vi "FpgaSession_GET.vi"(8 "error in":errorcluster, 11 "lia rt in":refnum<class "Lock-In Amplifier Example RT.lvclass">) -> (0 "error out":errorcluster, 2 "fpga interface":refnum<class "LIA Host Interface FPGA.lvclass">, 3 "lia rt out":refnum<class "Lock-In Amplifier Example RT.lvclass">)   [LabVIEW 2017, in "Lock-In Amplifier Example RT.lvclass"]
uses:
  Lock-In Amplifier Example RT.lvclass
  interface/Interface FPGA/LIA Host Interface FPGA.lvclass
  Lock-In Amplifier Example RT.lvclass/Lock-In Amplifier Example RT.ctl
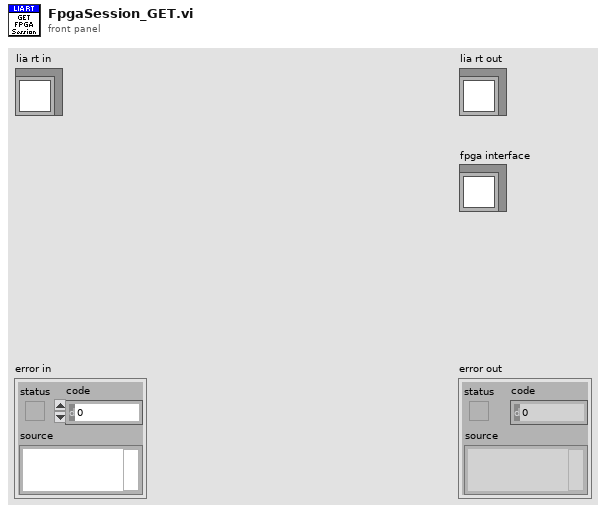
[diagram p1: front panel]
types:
  T1 = typedef "Lock-In Amplifier Example RT.lvclass/session data.ctl" = cluster{"server":refnum<class "RT FlexRIO Server TCP.lvclass">, "fpga interface":refnum<class "LIA Host Interface FPGA.lvclass">}
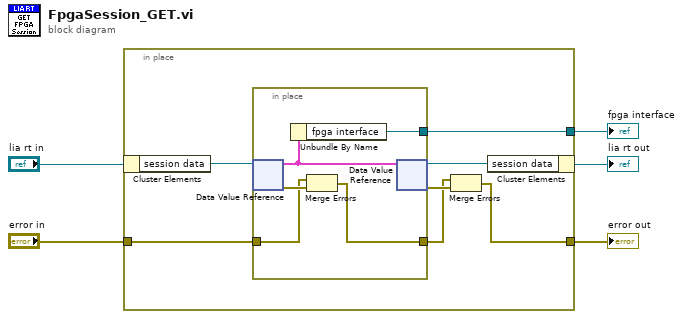
[diagram p0: block diagram]
diagram:
  n1 = in-place {
    in-place-border: "error in" -> [w10]
    in-place-border: [w7] -> w2
    in-place-border: [w6] -> w1
    n2 = in-place-cluster #1("lia rt in") -> ("session data"=w12:refnum<data-value>)
    n3 = in-place {
      in-place-border: w10 -> [w15]
      in-place-border: [w14] -> w8
      in-place-border: [w13] -> w6
      n4 = in-place-dvr #2(w12) -> (w17:T1, w16:errorcluster)
      n5 = Unbundle By Name(w17) -> ("fpga interface"=w13:refnum<class "LIA Host Interface FPGA.lvclass">)
      n6 = Merge Errors(w15, w16) -> (w14:errorcluster)
      n7 = in-place-dvr #2(w17) -> (w11:refnum<data-value>, w9:errorcluster)
    }
    n8 = Merge Errors(w8, w9) -> (w7:errorcluster)
    n9 = in-place-cluster #1("session data"=w11) -> (→"lia rt out":refnum<class "Lock-In Amplifier Example RT.lvclass">)
  }
  "error out" <- w2
  "fpga interface" <- w1
